vi "deleteUpdateTime.vi"(8 "error in (no error)":errorcluster, 11 "ScriptEventList in":refnum<class "ScriptEventList.lvclass">) -> (0 "error out":errorcluster, 3 "ScriptEventList out":refnum<class "ScriptEventList.lvclass">)   [LabVIEW 2011, in "Tools.lvlib" / "Scripting.lvlib" / "ScriptEventList.lvclass"]
uses:
  ScriptEventList.lvclass
  ScriptEventList.lvclass/ScriptEventList.ctl
  ScriptEvent.lvclass
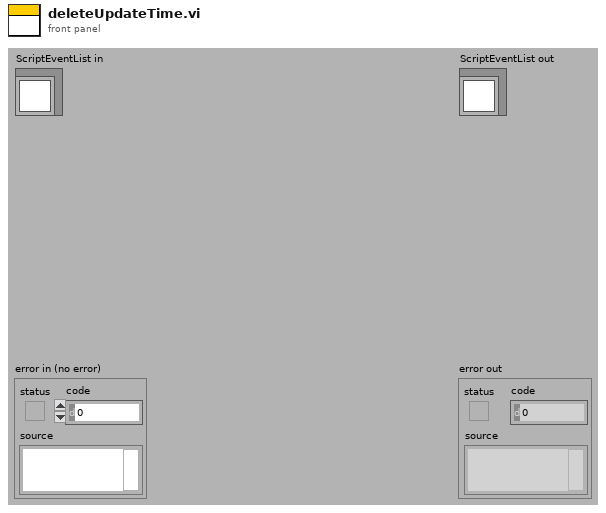
[diagram p1: front panel]
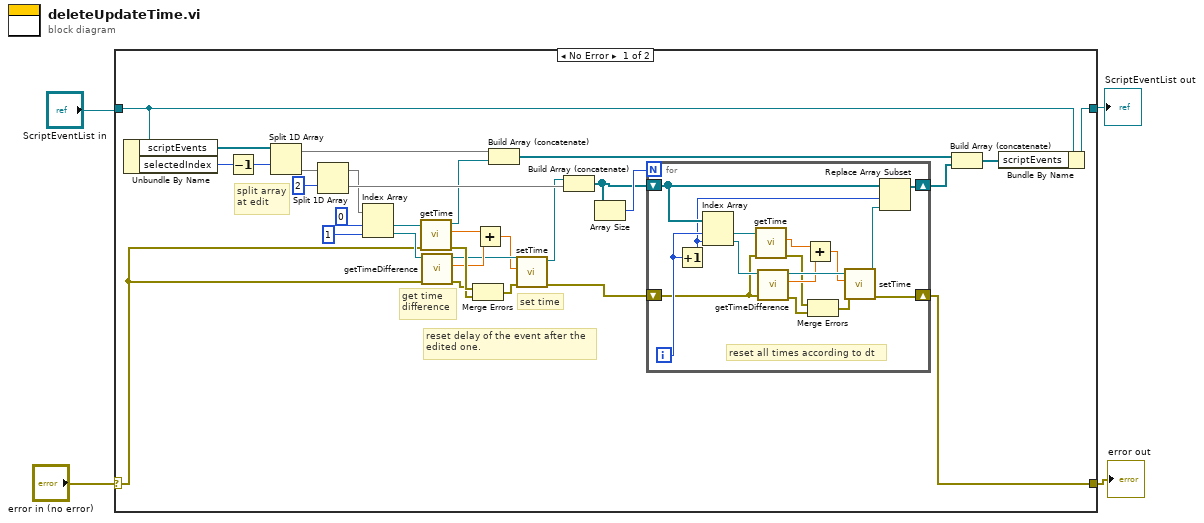
[diagram p0: block diagram]
diagram:
  n1 = case shown="No Error" "error in (no error)" {
    selector: "error in (no error)" -> [w14 w53]
    tunnel: [w17 w53] -> w2
    tunnel: [w18 w52] -> w1
    tunnel: "ScriptEventList in" -> [w19 w52]
    frame No Error {
      # "reset delay of the event after the\nedited one."
      # "split array\nat edit"
      # "set time"
      # "get time\ndifference"
      n2 = Unbundle By Name(w19) -> ("scriptEvents"=w33:refnum<class "ScriptEvent.lvclass">[], "selectedIndex"=w35:i32)
      n3 = Decrement(x=w35) -> (x-1=w34:i32)
      n4 = Split 1D Array(array=w33, index=w34) -> (first subarray=w28:refnum<class "ScriptEvent.lvclass">[], second subarray=w32:refnum<class "ScriptEvent.lvclass">[])
      n5 = Split 1D Array(array=w32, index=2) -> (first subarray=w25:refnum<class "ScriptEvent.lvclass">[], second subarray=w26:refnum<class "ScriptEvent.lvclass">[])
      n6 = Index Array(array=w25, index #1=0, index #2=1) -> (element #1=w29:refnum<class "ScriptEvent.lvclass">, element #2=w15:refnum<class "ScriptEvent.lvclass">)
      n7 = call "getTime.vi"("error in (no error)"=w14, "ScriptEvent.lvclass in"=w29) -> ("error out"=w27:errorcluster, "time"=w12:dbl, "ScriptEvent.lvclass out"=w10:refnum<class "ScriptEvent.lvclass">)  [unwired: 7 in]
      n8 = call "getTimeDifference.vi"("error in (no error)"=w14, "ScriptEvent.lvclass in"=w15) -> ("error out"=w13:errorcluster, "time difference"=w11:dbl, "ScriptEvent.lvclass out"=w9:refnum<class "ScriptEvent.lvclass">)  [unwired: 7 in]
      n9 = Merge Errors(w27, w13) -> (w5:errorcluster)
      n10 = Add(x=w12, y=w11) -> (x+y=w7:dbl)
      n11 = Build Array (concatenate)(w28, w10) -> (w22:refnum<class "ScriptEvent.lvclass">[])
      n12 = call "setTime.vi"("error in (no error)"=w5, "time"=w7, "ScriptEvent.lvclass in"=w9) -> ("error out"=w6:errorcluster, "ScriptEvent.lvclass out"=w8:refnum<class "ScriptEvent.lvclass">)  [unwired: 7 in]
      n13 = Build Array (concatenate)(w8, w26) -> (w23:refnum<class "ScriptEvent.lvclass">[])
      n14 = Array Size(array=w23) -> (size(s)=w24:i32)
      n15 = for {
        N: w24 -> [_]
        shift-right: [w36] -> w21
        shift-left: w23 -> [w39]
        shift-right: [w40] -> w17
        shift-left: w6 -> [w48]
        i -> [w51]
        # "reset all times according to dt"
        n16 = Increment(x=w51) -> (x+1=w38:i32)
        n17 = Index Array(array=w39, index #1=w51, index #2=w38) -> (element #1=w50:refnum<class "ScriptEvent.lvclass">, element #2=w49:refnum<class "ScriptEvent.lvclass">)
        n18 = call "getTime.vi"("error in (no error)"=w48, "ScriptEvent.lvclass in"=w50) -> ("error out"=w43:errorcluster, "time"=w46:dbl)  [unwired: 7 in, 1 out]
        n19 = call "getTimeDifference.vi"("error in (no error)"=w48, "ScriptEvent.lvclass in"=w49) -> ("error out"=w42:errorcluster, "time difference"=w45:dbl, "ScriptEvent.lvclass out"=w47:refnum<class "ScriptEvent.lvclass">)  [unwired: 7 in]
        n20 = Add(x=w46, y=w45) -> (x+y=w44:dbl)
        n21 = Merge Errors(w43, w42) -> (w41:errorcluster)
        n22 = call "setTime.vi"("error in (no error)"=w41, "time"=w44, "ScriptEvent.lvclass in"=w47) -> ("error out"=w40:errorcluster, "ScriptEvent.lvclass out"=w37:refnum<class "ScriptEvent.lvclass">)  [unwired: 7 in]
        n23 = Replace Array Subset(array=w39, new element=w37, index=w38) -> (w36:refnum<class "ScriptEvent.lvclass">[])
      }
      n24 = Build Array (concatenate)(w22, w21) -> (w20:refnum<class "ScriptEvent.lvclass">[])
      n25 = Bundle By Name(cluster=w19, "scriptEvents"=w20) -> (w18:refnum<class "ScriptEventList.lvclass">)
    }
    frame Error {
    }
  }
  "error out" <- w2
  "ScriptEventList out" <- w1
